vi "Measuring Complete - AndreTec-5.vi"() -> ()   [LabVIEW 2014]
doc: "André Romero - 2016\nandretec@ifsc.usp.br\nIFSC - USP"
uses:
  <vilib>/Analysis/Matrix/Datatypes/RealMatrix.ctl
  C:/UserLabs/Andre/AutoLabView/04-07-2017/Autolab SDK 1.11/EcoChemie.Autolab.Sdk.dll
  EcoChemie.Autolab.Sdk.dll
  <vilib>/Instr/_visa.llb/VISA Configure Serial Port (Instr).vi
  <vilib>/Utility/file.llb/Write To Spreadsheet File (DBL).vi
  <vilib>/Analysis/Matrix/NI_Matrix.lvlib
panel:
  out "Procedure array":path[](array[path])=[path "C:/Users/user/Documents/My Procedures 1.11/Procedures/bla.nox", path "C:/Users/user/Documents/My Procedures 1.11/Procedures/bla2.nox", path "", path "", path "", path "", path "", path ""]
  in  "Tab Control":enum32{"Settings", "Measuring..."}(tab)
  in  "Load Procedure #8":path
  in  "Load Procedure #7":path
  in  "Load Procedure #6":path
  in  "Load Procedure #5":path
  in  "Load Procedure #4":path
  in  "Load Procedure #3":path
  in  "Load Procedure #2":path=path "C:/Users/user/Documents/My Procedures 1.11/Procedures/bla2.nox"
  in  "Load Procedure #1":path=path "C:/Users/user/Documents/My Procedures 1.11/Procedures/bla.nox"
  in  "Start Measurement":bool
  out "Measured data":cluster{"Y":dbl[], "Y":dbl[]}[](graph)=[{"Y"=[7.324218750000278e-05, 7.324218750000278e-05, 7.324218750000278e-05, 7.324218750000278e-05, 7.324218750000278e-05, 7.324218750000278e-05, 7.324218750000278e-05, 7.324218750000278e-05, 7.324218750000278e-05, 7.324218750000278e-05, 7.324218750000278e-05, 7.324218750000278e-05, 7.324218750000278e-05, 7.324218750000278e-05, 7.324218750000278e-05, 7.324218750000278e-05, 7.324218750000278e-05, 7.324218750000278e-05, 7.324218750000278e-05, 7.324218750000278e-05, 7.324218750000278e-05, 7.324218750000278e-05, 7.324218750000278e-05, 7.324218750000278e-05, 7.324218750000278e-05, 7.324218750000278e-05, 7.324218750000278e-05, 7.324218750000278e-05, 7.324218750000278e-05, 7.324218750000278e-05, 7.324218750000278e-05, 7.324218750000278e-05, 3.967285156250555e-05, 0.007351684570312503, 0.0195159912109375, 0.026904296874999997, 0.039157104492187504, 0.048931884765625, 0.06103515625, 0.068450927734375, 0.078125, 0.095245361328125, 0.10504150390625, 0.114776611328125, 0.1246337890625, 0.1343994140625, 0.144134521484375, 0.156402587890625, 0.163787841796875, 0.173431396484375, 0.185821533203125, 0.193084716796875, 0.205322265625, 0.215057373046875, 0.224945068359375, 0.234649658203125, 0.244384765625, 0.254180908203125, 0.266448974609375, 0.27386474609375, 0.285980224609375, 0.293365478515625, 0.30560302734375, 0.315277099609375, 0.32525634765625, 0.33502197265625, 0.347259521484375, 0.354461669921875, 0.364288330078125, 0.3765869140625, 0.38623046875, 0.396148681640625, 0.40594482421875, 0.415618896484375, 0.42791748046875, 0.435302734375, 0.447540283203125, 0.45477294921875, 0.467041015625, 0.474395751953125, 0.4864501953125, 0.4864501953125, 0.4864501953125, 0.4864501953125, 0.4864501953125, 0.4864501953125, 0.4864501953125, 0.4864501953125, 0.4864501953125, 0.4864501953125, 0.4864501953125, 0.4864501953125, 0.4864501953125, 0.4864501953125, 0.4864501953125, 0.4864501953125, 0.4864501953125, 0.4864501953125, 0.4864501953125, 0.4864501953125, 0.4864501953125, 0.4864501953125, 0.4864501953125, 0.4864501953125, 0.4864501953125, 0.4864501953125, 0.4864501953125, 0.4864501953125, 0.4864501953125, 0.4864501953125, 0.4864501953125, 0.4864501953125, 0.4864501953125, 0.4864501953125, 0.4864501953125, 0.4864501953125, 0.4864501953125, 0.4864501953125, 0.4864501953125, 0.4864501953125, 0.4864501953125, 0.4864501953125, 0.4864501953125, 0.4864501953125, 0.4864501953125, 0.4864501953125], "Y"=[-1.5228271484375027e-09, -1.5228271484375027e-09, -1.5228271484375027e-09, -1.5228271484375027e-09, -1.5228271484375027e-09, -1.5228271484375027e-09, -1.5228271484375027e-09, -1.5228271484375027e-09, -1.5228271484375027e-09, -1.5228271484375027e-09, -1.5228271484375027e-09, -1.5228271484375027e-09, -1.5228271484375027e-09, -1.5228271484375027e-09, -1.5228271484375027e-09, -1.5228271484375027e-09, -1.5228271484375027e-09, -1.5228271484375027e-09, -1.5228271484375027e-09, -1.5228271484375027e-09, -1.5228271484375027e-09, -1.5228271484375027e-09, -1.5228271484375027e-09, -1.5228271484375027e-09, -1.5228271484375027e-09, -1.5228271484375027e-09, -1.5228271484375027e-09, -1.5228271484375027e-09, -1.5228271484375027e-09, -1.5228271484375027e-09, -1.5228271484375027e-09, -1.5228271484375027e-09, 1.2298583984375e-09, 8.026123046875e-09, 2.056884765625e-08, 2.8045654296875e-08, 4.3182373046875e-08, 5.0750732421875e-08, 6.0791015625e-08, 7.302856445312499e-08, 8.0780029296875e-08, 9.7625732421875e-08, 1.02691650390625e-07, 1.1566162109375e-07, 1.23779296875e-07, 1.3873291015625e-07, 1.4031982421875e-07, 1.5744018554687499e-07, 1.6473388671875e-07, 1.7724609375e-07, 1.8524169921875e-07, 1.97265625e-07, 2.03948974609375e-07, 2.15118408203125e-07, 2.2833251953125e-07, 2.3315429687499998e-07, 2.47528076171875e-07, 2.5543212890624997e-07, 2.6641845703125e-07, 2.72979736328125e-07, 2.86376953125e-07, 2.97393798828125e-07, 3.0657958984375e-07, 3.16162109375e-07, 3.27911376953125e-07, 3.33251953125e-07, 3.4716796874999997e-07, 3.55987548828125e-07, 3.6611938476562497e-07, 3.74664306640625e-07, 3.900146484375e-07, 3.9682006835937497e-07, 4.1180419921874997e-07, 4.16595458984375e-07, 4.2974853515624997e-07, 4.3438720703125e-07, 4.505615234375e-07, 4.55657958984375e-07, 4.6716308593749996e-07, 4.7686767578125e-07, 4.91546630859375e-07, 4.91546630859375e-07, 4.91546630859375e-07, 4.91546630859375e-07, 4.91546630859375e-07, 4.91546630859375e-07, 4.91546630859375e-07, 4.91546630859375e-07, 4.91546630859375e-07, 4.91546630859375e-07, 4.91546630859375e-07, 4.91546630859375e-07, 4.91546630859375e-07, 4.91546630859375e-07, 4.91546630859375e-07, 4.91546630859375e-07, 4.91546630859375e-07, 4.91546630859375e-07, 4.91546630859375e-07, 4.91546630859375e-07, 4.91546630859375e-07, 4.91546630859375e-07, 4.91546630859375e-07, 4.91546630859375e-07, 4.91546630859375e-07, 4.91546630859375e-07, 4.91546630859375e-07, 4.91546630859375e-07, 4.91546630859375e-07, 4.91546630859375e-07, 4.91546630859375e-07, 4.91546630859375e-07, 4.91546630859375e-07, 4.91546630859375e-07, 4.91546630859375e-07, 4.91546630859375e-07, 4.91546630859375e-07, 4.91546630859375e-07, 4.91546630859375e-07, 4.91546630859375e-07, 4.91546630859375e-07, 4.91546630859375e-07, 4.91546630859375e-07, 4.91546630859375e-07, 4.91546630859375e-07, 4.91546630859375e-07]}]
  out "Autolab Connected":bool
  out "Blacklisted Commands detected":bool
  out "Y axis value":dbl=4.91546630859375e-07
  out "X axis value":dbl=0.4864501953125
  in  "X axis Signal":string(combo)="WE(1).Potential"
  in  "Y axis Signal":string(combo)="WE(1).Current"
  out "Points":i32=30
  out "Sensor":i32=2
  out "Measurement active":bool
  in  "Abort":bool
  in  "String":string="Wait !!!! Instrument is initializing ...."
  out "Measurement":cluster{dbl[], dbl[]}(graph)={[0.4864501953125, 0.4864501953125, 0.4864501953125, 0.4864501953125, 0.4864501953125, 0.4864501953125, 0.4864501953125, 0.4864501953125, 0.4864501953125, 0.4864501953125, 0.4864501953125, 0.4864501953125, 0.4864501953125, 0.4864501953125, 0.4864501953125, 0.4864501953125, 0.4864501953125, 0.4864501953125, 0.4864501953125, 0.4864501953125, 0.4864501953125, 0.4864501953125, 0.4864501953125, 0.4864501953125, 0.4864501953125, 0.4864501953125, 0.4864501953125, 0.4864501953125, 0.4864501953125, 0.4864501953125, 0.4864501953125], [4.91546630859375e-07, 4.91546630859375e-07, 4.91546630859375e-07, 4.91546630859375e-07, 4.91546630859375e-07, 4.91546630859375e-07, 4.91546630859375e-07, 4.91546630859375e-07, 4.91546630859375e-07, 4.91546630859375e-07, 4.91546630859375e-07, 4.91546630859375e-07, 4.91546630859375e-07, 4.91546630859375e-07, 4.91546630859375e-07, 4.91546630859375e-07, 4.91546630859375e-07, 4.91546630859375e-07, 4.91546630859375e-07, 4.91546630859375e-07, 4.91546630859375e-07, 4.91546630859375e-07, 4.91546630859375e-07, 4.91546630859375e-07, 4.91546630859375e-07, 4.91546630859375e-07, 4.91546630859375e-07, 4.91546630859375e-07, 4.91546630859375e-07, 4.91546630859375e-07, 4.91546630859375e-07]}
  out "error out":errorcluster
  out "VISA resource name out":refnum<visa-resource-name>="ASRL3::INSTR"
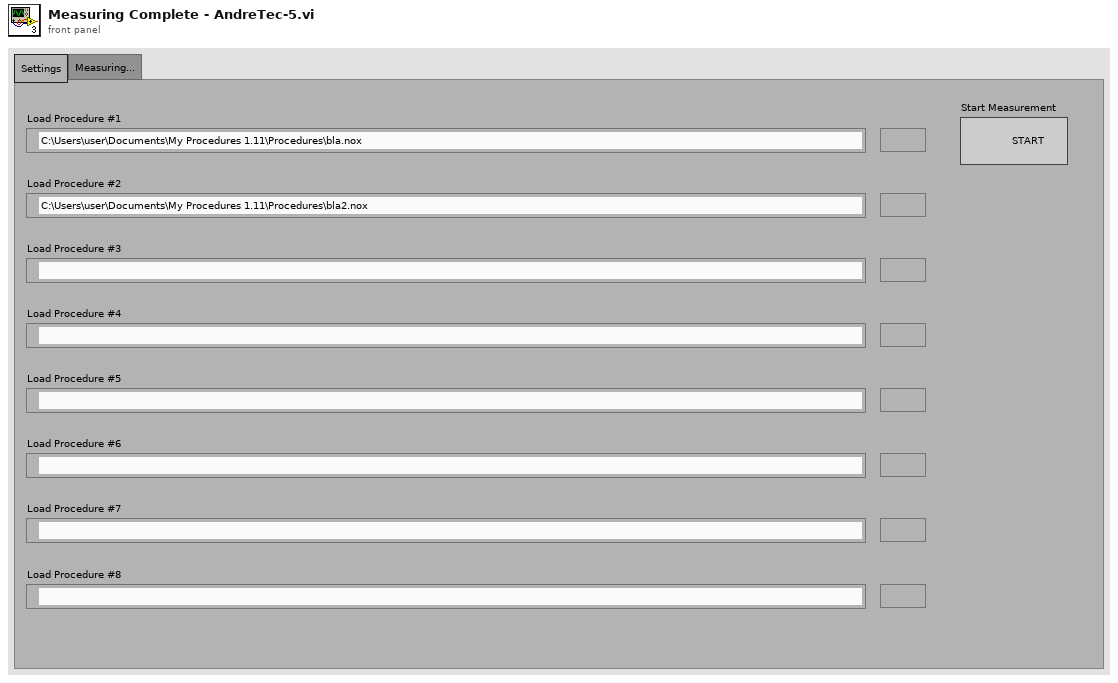
[diagram p1: front panel]
types:
  T1 = typedef "NI_Matrix.lvlib/RealMatrix.ctl" = dbl[][]
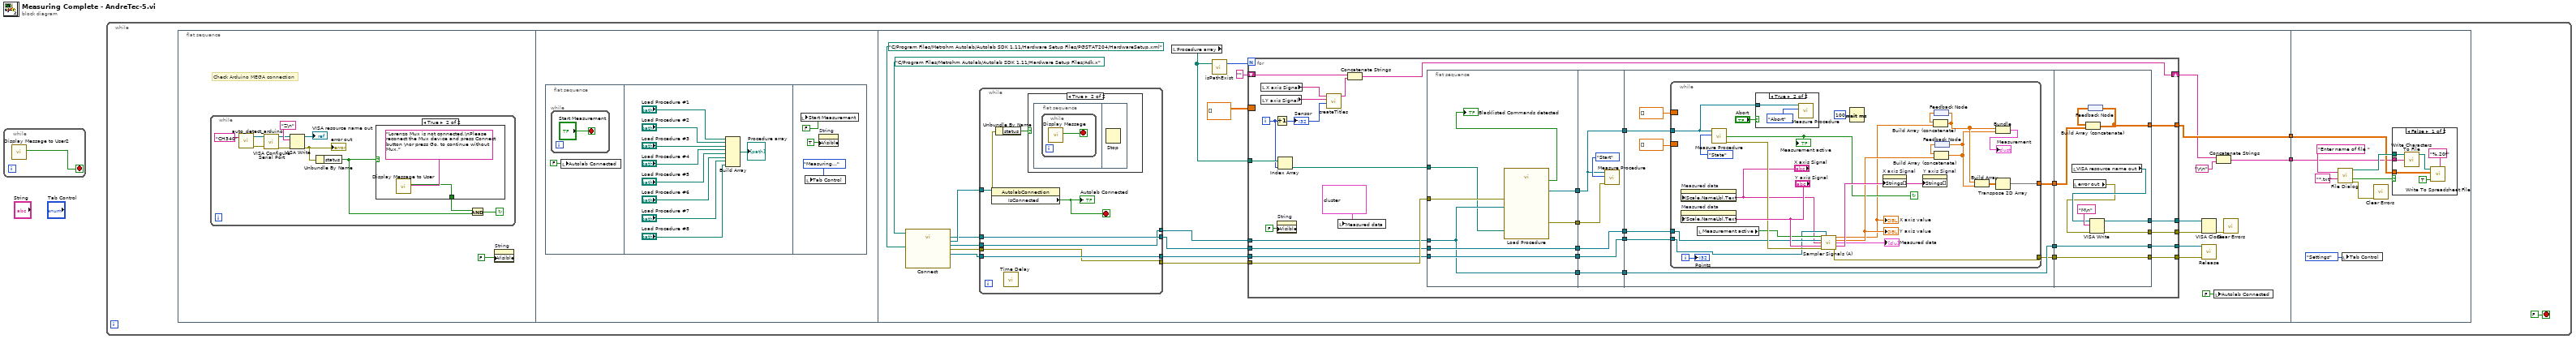
[diagram p0: block diagram]
diagram:
  n1 = while {
    stop <- w1 stop-if-true
    n2 = call "Display Message to User2"() -> ("OK"=w1:bool)  [unwired: 10 in, 1 out]
  }
  n3 = while {
    stop <- FALSE stop-if-true
    n4 = flat-sequence {
      tunnel: [w38] -> w3
      tunnel: [w36] -> w2
      tunnel: w3 -> [w159]
      tunnel: w2 -> [w158]
      frame #0 {
        # "Check Arduino MEGA connection"
        n5 = while {
          stop <- w8 continue-if-true
          n6 = call "auto_detect_arduino.vi"("instr name"="CH340") -> ("VISA resource name"=w16:refnum<visa-resource-name>, "error out"=w9:errorcluster)  [unwired: 1 in, 1 out]
          n7 = call-poly "VISA Configure Serial Port"("VISA resource name"=w16, "error in (no error)"=w9) -> ("VISA resource name out"=w13:refnum<visa-resource-name>, "error out"=w12:errorcluster)  [unwired: 7 in, 5 out]
          n8 = VISA Write(VISA resource name=w13, write buffer="Z\n" ("Command"), error in (no error)=w12) -> (VISA resource name out=→"VISA resource name out":refnum<visa-resource-name>, error out=w10:errorcluster)  [unwired: 1 out]
          "error out" <- w10
          n9 = Unbundle By Name(w10) -> ("status"=w7:bool)
          n10 = case shown="True" w7 {
            tunnel: [_ w17] -> w6
            frame False {
            }
            frame True {
              n11 = call "Display Message to User"("Message"="Lorenzo Mux is not connected.\nPlease reconect the Mux device and press Connect button \nor press Go, to continue without Mux.") -> ("Connect"=w17:bool)  [unwired: 9 in, 1 out]
            }
          }
          n12 = And(x=w6, y=w7) -> (x .and. y?=w8:bool)
        }
        n13 = property on="String" class="Str"("Visible"=FALSE) -> ()  [unwired: 2 in, 2 out]
      }
      frame #1 {
        n14 = flat-sequence {
          frame #0 {
            n15 = while {
              stop <- "Start Measurement" stop-if-true
            }
            n16 = local write "Autolab Connected"(FALSE ("Autolab Connected")) -> ()
          }
          frame #1 {
            n17 = Build Array("Load Procedure #1", "Load Procedure #2", "Load Procedure #3", "Load Procedure #4", "Load Procedure #5", "Load Procedure #6", "Load Procedure #7", "Load Procedure #8") -> (→"Procedure array":path[])
          }
          frame #2 {
            n18 = local write "Start Measurement"(FALSE ("Start Measurement")) -> ()
            n19 = local write "Tab Control"(enum32{"Settings", "Measuring..."}."Measuring..." ("Tab Control")) -> ()
            n20 = property on="String" class="Str"("Visible"=TRUE) -> ()  [unwired: 2 in, 2 out]
          }
        }
      }
      frame #2 {
        n21 = call "Connect.vi"("Embedded Exe File"=path "C:/Program Files/Metrohm Autolab/Autolab SDK 1.11/Hardware Setup Files/Adk.x", "Hardware Setup File"=path "C:/Program Files/Metrohm Autolab/Autolab SDK 1.11/Hardware Setup Files/PGSTAT204/HardwareSetup.xml") -> ("Sampler"=w54:refnum<k24>, "AutolabConnection"=w55:refnum<k24>, "instrument"=w52:refnum<k24>, "Ei"=w47:refnum<k24>, "error out"=w49:errorcluster)  [unwired: 1 in, 8 out]
        n22 = while {
          tunnel: w55 -> [w154]
          tunnel: w54 -> [w151]
          tunnel: [w151] -> w53
          tunnel: w52 -> [w150]
          tunnel: [w150] -> w51
          tunnel: w47 -> [w149]
          tunnel: [w149] -> w50
          tunnel: w49 -> [w148]
          tunnel: [w148] -> w48
          stop <- w155 stop-if-true
          n23 = property class="AutolabConnection"(reference=w154) -> (error out=w152:errorcluster, "IsConnected"=w155:bool)  [unwired: 1 in, 1 out]
          "Autolab Connected" <- w155
          n24 = Unbundle By Name(w152) -> ("status"=w153:bool)
          n25 = call "Time Delay"() -> ()  [unwired: 2 in, 10 out]
          n26 = case shown="True" w153 {
            frame False {
            }
            frame True {
              n27 = flat-sequence {
                frame #0 {
                  n28 = while {
                    stop <- w156 stop-if-true
                    n29 = call "Display Message"() -> ("OK"=w156:bool)  [unwired: 10 in, 1 out]
                  }
                }
                frame #1 {
                  n30 = Stop() -> ()  [unwired: 1 in]
                }
              }
            }
          }
        }
        n31 = local read "Procedure array"() -> (w33:path[])
        n32 = call "isPathExist.vi"("Array"=w33) -> ("Numeric"=w34:i16)  [unwired: 2 in]
        n33 = for {
          N: w34 -> [_]
          tunnel: [w78] -> w46
          tunnel: [w77] -> w45
          tunnel: [w76] -> w43
          tunnel: [w75] -> w42
          tunnel: w48 -> [w74]
          tunnel: w51 -> [w73]
          tunnel: w53 -> [w72]
          tunnel: w50 -> [w71]
          tunnel: [w69] -> w38
          border: T1 [] ("Real Matrix") -> [_]
          shift-right: [w66] -> w37
          shift-left: "" -> [w67]
          tunnel: w33 -> [w61]
          i -> [w60]
          n34 = local read "Y axis Signal"() -> (w64:string)
          n35 = local read "X axis Signal"() -> (w65:string)
          n36 = Increment(x=w60) -> (x+1=w63:i32)
          "Sensor" <- w63
          n37 = property on="String" class="Str"("Visible"=FALSE) -> ()  [unwired: 2 in, 2 out]
          n38 = Index Array(array=w61, index=w60) -> (element=w59:path)
          n39 = call "createTitles.vi"("Numeric"=w63, "Y axis Signal"=w64, "X axis Signal"=w65) -> ("String"=w62:string)  [unwired: 8 in]
          n40 = local write "Measured data"(cluster{"Y":dbl[], "Y":dbl[]}[] [{"Y"=array[2393 elements], "Y"=array[2393 elements]}] ("Measured data")) -> ()
          n41 = Concatenate Strings(w67, w62) -> (w66:string)
          n42 = flat-sequence {
            tunnel: [w96] -> w89
            tunnel: [w95] -> w88
            tunnel: [w93] -> w87
            tunnel: [w92] -> w86
            tunnel: [w91] -> w85
            tunnel: w73 -> [w91]
            tunnel: w74 -> [w94]
            tunnel: w72 -> [w93]
            tunnel: w71 -> [w92]
            tunnel: w59 -> [w90]
            tunnel: w89 -> [w101]
            tunnel: w88 -> [w102]
            tunnel: [w101] -> w84
            tunnel: w87 -> [w100]
            tunnel: w86 -> [w99]
            tunnel: [w100] -> w83
            tunnel: [w99] -> w82
            tunnel: [w98] -> w81
            tunnel: w85 -> [w98]
            tunnel: w84 -> [w111]
            tunnel: w83 -> [w110]
            tunnel: w82 -> [w109]
            tunnel: w81 -> [w108]
            tunnel: [w108] -> w80
            tunnel: [w104] -> w79
            tunnel: [w107] -> w70
            tunnel: w80 -> [w147]
            tunnel: w79 -> [w146]
            tunnel: [w147] -> w78
            tunnel: [w146] -> w77
            tunnel: [w142] -> w76
            tunnel: [w141] -> w75
            tunnel: w70 -> [w140]
            tunnel: [w138] -> w69
            frame #0 {
              n43 = call "Load Procedure.vi"("error in (no error)"=w94, "Procedure"=w90, "Instrument"=w91) -> ("error out"=w95:errorcluster, "Contains"=→"Blacklisted Commands detected":bool, "LoadProcedure"=w96:refnum<k24>)  [unwired: 6 out]
            }
            frame #1 {
              n44 = call "Measure Procedure.vi"("error in"=w102, "Request for procedure"=enum16{"State", "Save", "Abort", "Start"}."Start", "LoadProcedure"=w101) -> ()  [unwired: 1 in, 8 out]
            }
            frame #2 {
              n45 = while {
                tunnel: w111 -> [w128]
                tunnel: w110 -> [w129]
                tunnel: w109 -> [w113]
                tunnel: [w116] -> w107
                border: dbl[] [] -> [_]
                border: dbl[] [] -> [_]
                tunnel: [w115] -> w104
                i -> [w125]
                stop <- w120 continue-if-true
                n46 = property on="Measured data" class="XYGraph (strict)"("XScale.NameLbl.Text"="X axis Signal") -> ()  [unwired: 2 in, 2 out]
                n47 = property on="Measured data" class="XYGraph (strict)"("YScale.NameLbl.Text"="Y axis Signal") -> ()  [unwired: 2 in, 2 out]
                n48 = local read "Measurement active"() -> (w131:bool)
                n49 = call "Measure Procedure.vi"("Request for procedure"=enum16{"State", "Save", "Abort", "Start"}."State", "LoadProcedure"=w128) -> ("error out"=w132:errorcluster, "IsMeasuring"=w120:bool)  [unwired: 2 in, 6 out]
                "Measurement active" <- w120
                n50 = case shown="True" "Abort" {
                  tunnel: w128 -> [_ w136]
                  frame False {
                  }
                  frame True {
                    n51 = call "Measure Procedure.vi"("Request for procedure"=enum16{"State", "Save", "Abort", "Start"}."Abort", "LoadProcedure"=w136) -> ()  [unwired: 2 in, 8 out]
                  }
                }
                n52 = call "Sampler Signals (A).vi"("IsMeasuring"=w131, "EI"=w113, "Sampler"=w129, "Signal X"="X axis Signal", "Signal Y"="Y axis Signal", "error in"=w132) -> ("X"=w114:dbl, "Y"=w122:dbl, "XY Graph"=→"Measured data":cluster{"Y":dbl[], "Y":dbl[]}[], "GetSignals"=w134:string[], "error out"=w115:errorcluster)  [unwired: 4 in, 1 out]
                "Y axis value" <- w122
                "X axis value" <- w114
                n53 = Wait (ms)(milliseconds to wait=u32 100) -> ()  [unwired: 1 out]
                n54 = property on="X axis Signal" class="CmbBox"("Strings[]"=w134) -> ()  [unwired: 2 in, 2 out]
                n55 = property on="Y axis Signal" class="CmbBox"("Strings[]"=w134) -> ()  [unwired: 2 in, 2 out]
                n56 = feedback #1() -> (w124:dbl[])
                n57 = Build Array (concatenate)(w124, w114) -> (w118:dbl[])
                n58 = feedback-in #1(w118) -> ()
                n59 = feedback #2() -> (w123:dbl[])
                n60 = Build Array (concatenate)(w123, w122) -> (w117:dbl[])
                n61 = feedback-in #2(w117) -> ()
                n62 = Build Array(w118, w117) -> (w119:dbl[][])
                n63 = Bundle(w118, w117) -> (→"Measurement":cluster{dbl[], dbl[]})  [unwired: 1 in]
                n64 = Transpose 2D Array(2D array=w119) -> (transposed array=w116:dbl[][])
                "Points" <- w125
              }
            }
            frame #3 {
              n65 = local read "VISA resource name out"() -> (w144:refnum<visa-resource-name>)
              n66 = local read "error out"() -> (w143:errorcluster)
              n67 = feedback #3() -> (w139:T1)
              n68 = Build Array (concatenate)(w139, w140) -> (w138:T1)
              n69 = feedback-in #3(w138) -> ()
              n70 = VISA Write(VISA resource name=w144, write buffer="M\n" ("Command"), error in (no error)=w143) -> (VISA resource name out=w142:refnum<visa-resource-name>, error out=w141:errorcluster)  [unwired: 1 out]
            }
          }
        }
        n71 = call "Release.vi"("error in (no error)"=w45, "Instrument"=w46) -> ()  [unwired: 1 in, 9 out]
        n72 = VISA Close(VISA resource name=w43, error in (no error)=w42) -> (error out=w44:errorcluster)
        n73 = local write "Autolab Connected"(FALSE ("Autolab Connected")) -> ()
        n74 = Concatenate Strings(w37, "\r\n") -> (w36:string)
        n75 = call <vilib>:"Clear Errors.vi"("error in (no error)"=w44) -> ()  [unwired: 5 in, 2 out]
      }
      frame #3 {
        n76 = call "File Dialog"("prompt"="Enter name of file ", "pattern (all files)"="*.txt") -> ("selected path"=w162:path, "cancelled"=w160:bool, "error out"=w161:errorcluster)  [unwired: 10 in, 1 out]
        n77 = local write "Tab Control"(enum32{"Settings", "Measuring..."}."Settings" ("Tab Control")) -> ()
        n78 = call <vilib>:"Clear Errors.vi"("error in (no error)"=w161) -> ()  [unwired: 5 in, 2 out]
        n79 = case shown="False" w160 {
          tunnel: w162 -> [w170 _]
          tunnel: w159 -> [w167 _]
          tunnel: w158 -> [w166 _]
          frame False {
            n80 = call <vilib>:"Write Characters To File.vi"("character string"=w166, "file path (dialog if empty)"=w170) -> ("new file path (Not A Path if cancelled)"=w169:path)  [unwired: 3 in]
            n81 = call-poly <vilib>:"Write To Spreadsheet File.vi"("format (%.3f)"="%.20f", "append to file? (new file:F)"=TRUE, "2D data"=w167, "file path (dialog if empty)"=w169) -> ()  [unwired: 4 in, 1 out]
          }
          frame True {
          }
        }
      }
    }
  }
